vi "EMS CID File Received.vi"(8 "error in (no error)":errorcluster, 10 "File Name":string, 11 "Master Controller in":refnum<class "Master Controller.lvclass">) -> (0 "error out":errorcluster, 3 "Master Controller out":refnum<class "Master Controller.lvclass">)   [LabVIEW 2015, in "Master Controller Core.lvlib" / "Master Controller.lvclass"]
uses:
  Master Controller.lvclass
  Communications/SCADA Communcations Actor/SCADA Communications/Controls/EMS Message Cluster.ctl
  <vilib>/ActorFramework/Message Enqueuer/Message Priority.ctl
  Master Controller.lvclass/Master Controller.ctl
  Communications/SCADA Communcations Actor/SCADA Communications Messages/Transmit EMS Message Msg/Transmit EMS Message Msg.lvclass/Transmit EMS Message Msg.ctl
  <vilib>/ActorFramework/Message Enqueuer/Message Enqueuer.lvclass/Message Enqueuer.ctl
  <vilib>/ActorFramework/Message Enqueuer/Enqueue.vi
  <vilib>/ActorFramework/Message Priority Queue/Priority Enqueue.vi
  Communications/SCADA Communcations Actor/SCADA Communications Messages/Transmit EMS Message Msg/Transmit EMS Message Msg.lvclass
  Communications/SCADA Communcations Actor/SCADA Communications/SCADA Communications.lvclass
  Utilities/Message Strings.llb/Message String Utilities.lvlib
  <vilib>/ActorFramework/Message Enqueuer/Message Enqueuer.lvclass
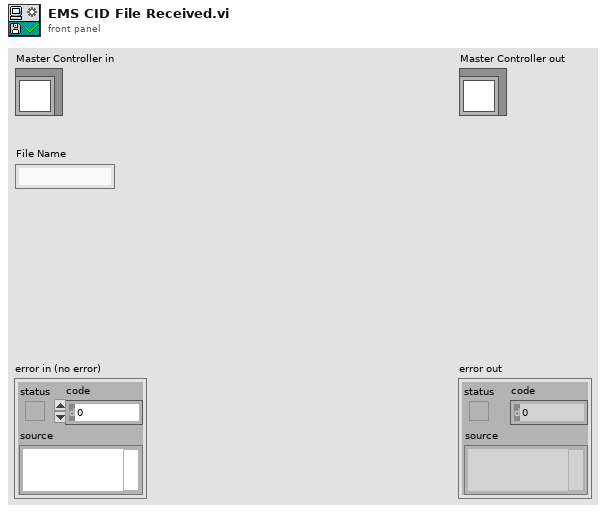
[diagram p1: front panel]
types:
  T1 = typedef "Actor Framework.lvlib/Message Enqueuer.lvclass/Message Priority.ctl" = enum16{"Low", "Normal", "High"}
  T2 = typedef "SCADA Communcations Actor.lvlib/SCADA Communications.lvclass/EMS Message Cluster.ctl" = cluster{"Name":string, "Content":string}
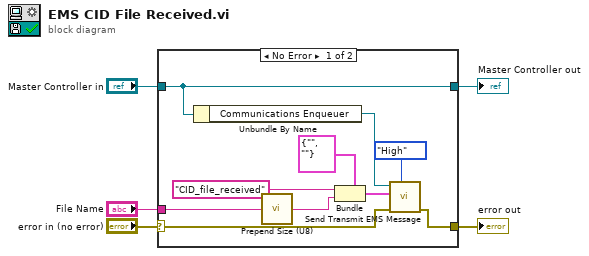
[diagram p0: block diagram]
diagram:
  n1 = case shown="No Error" "error in (no error)" {
    selector: "error in (no error)" -> [w9 w17]
    tunnel: [w11 w17] -> w4
    tunnel: [w15 w16] -> w2
    tunnel: "Master Controller in" -> [w15 w16]
    tunnel: "File Name" -> [w10 _]
    frame No Error {
      n2 = Unbundle By Name(w15) -> ("Communications Enqueuer"=w14:refnum<class "Message Enqueuer.lvclass">)
      n3 = call "Prepend Size (U8).vi"("String in"=w10) -> ("String out"=w8:string)
      n4 = Bundle(cluster=T2 {"Name"="", "Content"=""} ("Message"), "Name"="CID_file_received", "Content"=w8) -> (w12:T2)
      n5 = call "Send Transmit EMS Message.vi"("Message Priority (Normal)"=Message_Priority."High", "error in (no error)"=w9, "Message"=w12, "Message Enqueuer"=w14) -> ("error out"=w11:errorcluster)  [unwired: 6 in, 1 out]
    }
    frame Error {
    }
  }
  "error out" <- w4
  "Master Controller out" <- w2
